vi "DeSerializeMethod.vi"(0 "object in":refnum<class "JSONJDP.lvclass">, 2 "JSON":string, 5 "error in (no error)":errorcluster) -> (14 "object out":refnum<class "JSONJDP.lvclass">, 15 "Class":string, 16 "Method":string, 17 "Inputsstring":string, 19 "error out":errorcluster)   [LabVIEW 2018, in "JSONJDP.lvclass"]
uses:
  JSONJDP.lvclass
  6182dd3a-afaa-4f62-8a09-f3c3b357afd3.vi
  6df423e3-3664-47a8-bbce-bb948de1a9a3.vi
  <vilib>/JDP Science/JSONtext/JSON text to Variant.vi
  <vilib>/JDP Science/JSONtext/LVClass Serializer/JSONtext LVClass Serializer.lvclass
panel:
  out "error out 2":errorcluster
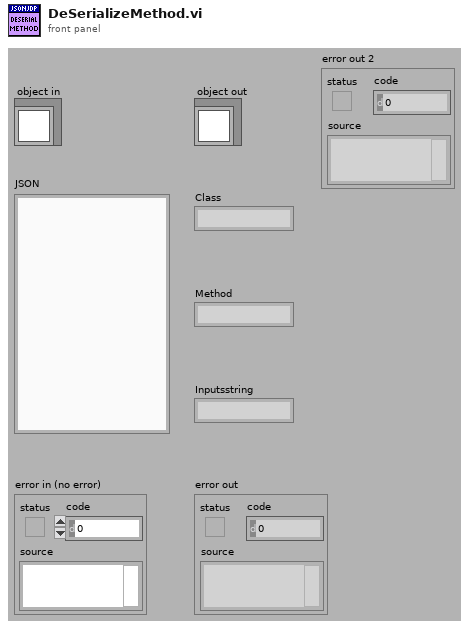
[diagram p1: front panel]
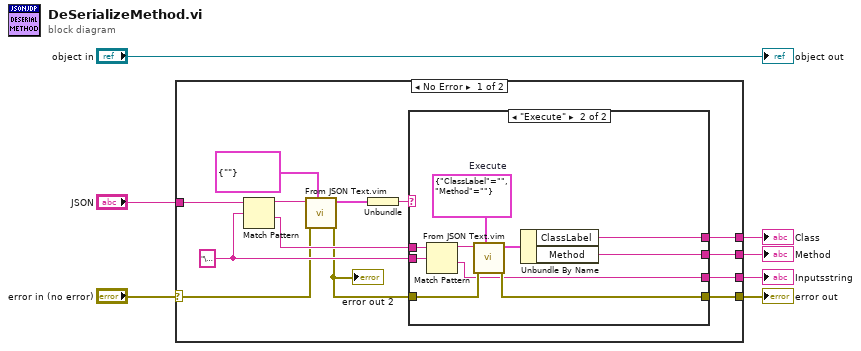
[diagram p0: block diagram]
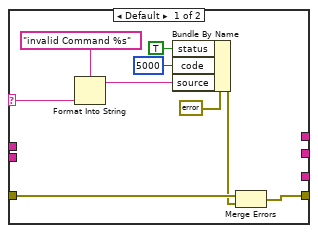
[diagram p2: hidden frame]
diagram:
  n1 = case shown="No Error" "error in (no error)" {
    selector: "error in (no error)" -> [w10 w40]
    tunnel: [w16 w40] -> w6
    tunnel: "JSON" -> [w17 _]
    tunnel: [w15 _] -> w2
    tunnel: [w14 _] -> w3
    tunnel: [w8 _] -> w1
    frame No Error {
      w18 = "\u0017" ("Delimiter")
      n2 = Match Pattern(string=w17, regular expression=w18) -> (before substring=w13:string, after substring=w20:string)  [unwired: 1 in, 2 out]
      n3 = call "From JSON Text.vim"("Data Type and Default Value"=cluster{"Command":string} {"Command"=""} ("output cluster"), "error in (no error)"=w10, "JSON"=w13) -> ("error out"=w9:errorcluster, "Data out"=w11:cluster{"Command":string})  [unwired: 7 in]
      "error out 2" <- w9
      n4 = Unbundle(w11) -> ("Command"=w19:string)
      n5 = case shown="\"Execute\"" w19 {
        selector: w19 -> [w25 _]
        tunnel: w20 -> [_ w39]
        tunnel: w9 -> [w28 w33]
        tunnel: w18 -> [_ w38]
        tunnel: [w29 w31] -> w16
        tunnel: [_ w37] -> w15
        tunnel: [_ w36] -> w14
        tunnel: [_ w30] -> w8
        frame Default {
          n6 = Format Into String(format string="invalid Command %s", w25) -> (resulting string=w23:string)  [unwired: 2 in, 1 out]
          n7 = Bundle By Name(cluster=errorcluster {"status"=TRUE, "code"=5000, "source"="invalid Commnad"} ("error in"), "status"=TRUE, "code"=5000, "source"=w23) -> (w24:errorcluster)
          n8 = Merge Errors(w28, w24) -> (w29:errorcluster)
        }
        frame "Execute" {
          w35 = cluster{"ClassLabel":string, "Method":string} {"ClassLabel"="", "Method"=""}  # Execute
          n9 = Match Pattern(string=w39, regular expression=w38) -> (before substring=w34:string, after substring=w30:string)  [unwired: 1 in, 2 out]
          n10 = call "From JSON Text.vim"("Data Type and Default Value"=w35, "error in (no error)"=w33, "JSON"=w34) -> ("error out"=w31:errorcluster, "Data out"=w32:cluster{"ClassLabel":string, "Method":string})  [unwired: 7 in]
          n11 = Unbundle By Name(w32) -> ("ClassLabel"=w37:string, "Method"=w36:string)
        }
      }
    }
    frame Error {
    }
  }
  "error out" <- w6
  "Class" <- w2
  "Method" <- w3
  "Inputsstring" <- w1
  "object out" <- "object in"
